vi "FileSystemWatcher.vi"(0 "Folder Path":path, 5 "error in (no error)":errorcluster caption="错误输入（无错误）", 7 "Filter":string) -> (14 "RegEvent":refnum<event-registration>, 19 "error out":errorcluster caption="错误输出")   [LabVIEW 2013]
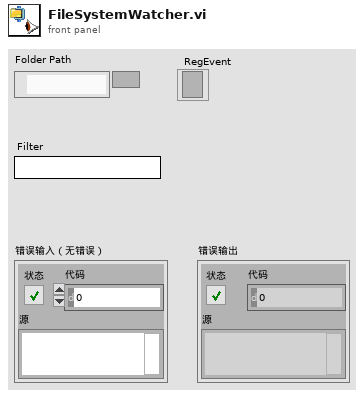
[diagram p1: front panel]
types:
  T1 = cluster{"ChangeType":i32, "FullPath":string, "Name":string, "OldFullPath":string, "OldName":string}
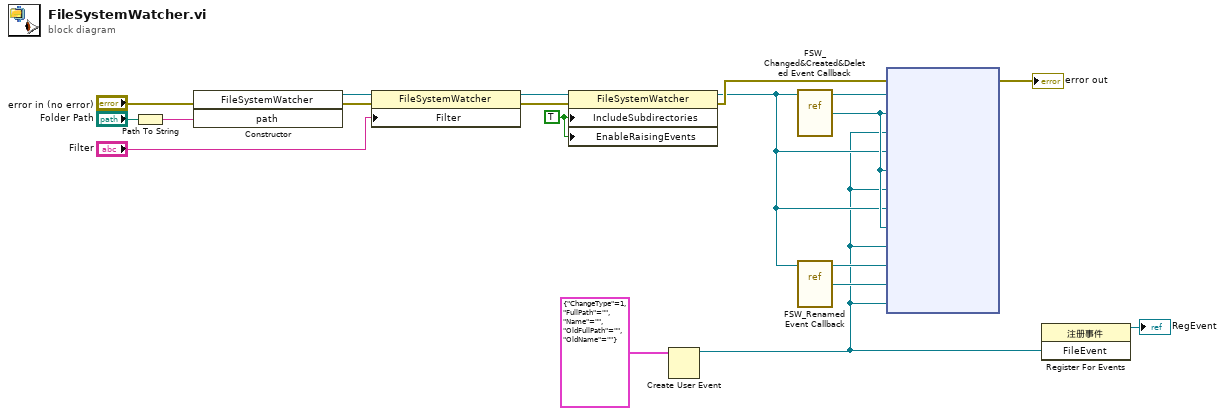
[diagram p0: block diagram]
diagram:
  w15 = TRUE ("IncludeSubdirectories")
  n1 = Path To String(path="Folder Path") -> (string=w16:string)
  n2 = constructor class="FileSystemWatcher"(error in="error in (no error)", "path"=w16) -> (reference out=w2:refnum<k24>, error out=w4:errorcluster)  [unwired: 2 in, 2 out]
  n3 = property on="属性节点" class="FileSystemWatcher"(reference=w2, error in=w4, "Filter"="Filter") -> (reference out=w5:refnum<k24>, error out=w3:errorcluster)
  n4 = property on="属性节点" class="FileSystemWatcher"(reference=w5, error in=w3, "IncludeSubdirectories"=w15, "EnableRaisingEvents"=w15) -> (reference out=w11:refnum<k24>, error out=w14:errorcluster)
  n5 = Create User Event(user event datatype=T1 {"ChangeType"=1, "FullPath"="", "Name"="", "OldFullPath"="", "OldName"=""} ("FileEvent")) -> (user event=w7:refnum<user-event>)  [unwired: 1 in, 1 out]
  n6 = vi-ref "FSW_Changed&Created&Deleted Event Callback.vi"() -> ("vi reference"=w12:refnum<vi>)
  n7 = vi-ref "FSW_Renamed Event Callback.vi"() -> ("vi reference"=w10:refnum<vi>)
  n8 = node(w14, w11, w12, w7, w11, w12, w7, w11, w12, w7, w11, w10, w7) -> (→"error out":errorcluster)  [unwired: 1 in, 1 out]
  n9 = register-events(w7) -> (reference out=→"RegEvent":refnum<event-registration>)  [unwired: 2 in, 1 out]
